vi "HFRR ADV v021 new software.vi"() -> ()   [LabVIEW 2025] (continued)
            n322 = property on="Password 3" class="Clust (strict)"("Visible"=TRUE) -> ()  [unwired: 2 in, 2 out]
            n323 = property on="Service Password Log" class="Str"("Visible"=TRUE) -> ()  [unwired: 2 in, 2 out]
          }
        }
      }
      event "Password 3.Service Password": Value Change {
        n324 = event-data() -> ()  [unwired: 1 in, 6 out]
        n325 = Unbundle By Name("Password 3") -> ("Service Password"=w417:string)
        n326 = call <vilib>:"Trim Whitespace.vi"("string"=w417) -> ("trimmed string"=w415:string)  [unwired: 1 in]
        n327 = Equal?(x=w415, y="Service@123") -> (x = y?=w416:bool)
        n328 = case shown="False" w416 {
          selector: w416 -> [w421 w423]
          frame False {
            n329 = local write "Service Password enable"(w421) -> ()
            n330 = property on="Service Password Log" class="Str"("Visible"=TRUE) -> ()  [unwired: 2 in, 2 out]
            n331 = property on="Tab Control 5" class="TabCtl (strict)"("Tabs Visible?"=TRUE ("Page Labels Display Visible?")) -> ()  [unwired: 2 in, 2 out]
          }
          frame True {
            n332 = property on="Service Password Log" class="Str"("Visible"=FALSE) -> ()  [unwired: 2 in, 2 out]
            "Service Password enable" <- w423
          }
        }
      }
      event "Sign In": Value Change {
        w425 = FALSE ("Visible")
        n333 = event-data() -> ()  [unwired: 1 in, 6 out]
        n334 = property on="About" class="Clust (strict)"("Visible"=w425) -> ()  [unwired: 2 in, 2 out]
        n335 = property on="Password 3" class="Clust (strict)"("Visible"=w425) -> ()  [unwired: 2 in, 2 out]
        n336 = property on="Service Password Log" class="Str"("Visible"=FALSE) -> ()  [unwired: 2 in, 2 out]
      }
      event "Info": Value Change {
        n337 = event-data() -> ()  [unwired: 1 in, 6 out]
        n338 = local read "Info"() -> (w427:bool)
        n339 = case shown="False" w427 {
          frame False {
            n340 = property on="About" class="Clust (strict)"("Visible"=FALSE) -> ()  [unwired: 2 in, 2 out]
          }
          frame True {
            n341 = property on="About" class="Clust (strict)"("Visible"=TRUE) -> ()  [unwired: 2 in, 2 out]
          }
        }
      }
      event "Calibration": Value Change {
        n342 = event-data() -> ()  [unwired: 1 in, 6 out]
        n343 = local read "Calibration"() -> (w431:bool)
        n344 = case shown="False" w431 {
          frame False {
            n345 = property on="Calibration 2" class="TabCtl (strict)"("Visible"=FALSE) -> ()  [unwired: 2 in, 2 out]
            n346 = local write "Cal Password"("" ("Cal Password")) -> ()
          }
          frame True {
            n347 = property on="Calibration 2" class="TabCtl (strict)"("Visible"=TRUE) -> ()  [unwired: 2 in, 2 out]
            n348 = local write "Cal Password"("" ("Cal Password")) -> ()
          }
        }
        n349 = property on="Wrong Password" class="Str"("Visible"=FALSE) -> ()  [unwired: 2 in, 2 out]
      }
      event "Cal Password": Value Change {
        n350 = event-data() -> ()  [unwired: 1 in, 6 out]
        n351 = local read "Cal Password"() -> (w439:string)
        n352 = call <vilib>:"Trim Whitespace.vi"("string"=w439) -> ("trimmed string"=w438:string)  [unwired: 1 in]
        n353 = Equal?(x=w438, y="Cal@321") -> (x = y?=w436:bool)
        n354 = case shown="True" w436 {
          frame False {
            n355 = property on="Wrong Password" class="Str"("Visible"=TRUE) -> ()  [unwired: 2 in, 2 out]
          }
          frame True {
            n356 = property on="Wrong Password" class="Str"("Visible"=FALSE) -> ()  [unwired: 2 in, 2 out]
            n357 = local write "Main Tab"(T2."About" ("Main Tab")) -> ()
            n358 = local write "Cal Password"("" ("Cal Password")) -> ()
            n359 = local write "Main Dashboard Buttons"(T1."About" ("Main Dashboard Buttons")) -> ()
            n360 = local write "Tab Control 5"(T12."Temperature Calibration" ("Tab Control 5")) -> ()
            n361 = property on="Calibration 2" class="TabCtl (strict)"("Visible"=FALSE) -> ()  [unwired: 2 in, 2 out]
            n362 = property on="Tab Control 5" class="TabCtl (strict)"("Tabs Visible?"=FALSE ("Page Labels Display Visible?")) -> ()  [unwired: 2 in, 2 out]
            n363 = local write "Calibration"(FALSE ("Calibration")) -> ()
          }
        }
      }
      event "Calibration Selection": Value Change {
        n364 = event-data() -> ()  [unwired: 1 in, 6 out]
        n365 = local read "Calibration Selection"() -> (w450:T8)
        n366 = case shown="\"Stroke Calibration\"" w450 {
          tunnel: [T7."Stroke" ("Main Calibration Tab") T7."Friction" ("Main Calibration Tab") T7."Main" ("Main Calibration Tab") T7."Temperature" ("Main Calibration Tab")] -> w449
          frame "Stroke Calibration" {
          }
          frame "Friction Force Calibration" {
          }
          frame Default {
          }
          frame "Temperature Calibration" {
          }
        }
        n367 = local write "Main Calibration Tab"(w449) -> ()
      }
      event "Back Stroke": Value Change {
        n368 = event-data() -> ()  [unwired: 1 in, 6 out]
        n369 = local write "Main Stroke Tab"(T9."Step 1" ("Main Stroke Tab")) -> ()
        n370 = local write "Main Calibration Tab"(T7."Main" ("Main Calibration Tab")) -> ()
        n371 = local write "Back Stroke"(FALSE ("Back Stroke")) -> ()
      }
      event "Step 2 Back": Value Change {
        n372 = event-data() -> ()  [unwired: 1 in, 6 out]
        n373 = local write "Main Stroke Tab"(T9."Step 1" ("Main Stroke Tab")) -> ()
        n374 = local write "Step 2 Back"(FALSE ("Back Stroke")) -> ()
      }
      event "Step 3 Back": Value Change {
        n375 = event-data() -> ()  [unwired: 1 in, 6 out]
        n376 = local write "Main Stroke Tab"(T9."Step 2" ("Main Stroke Tab")) -> ()
        n377 = local write "Step 3 Back"(FALSE ("Back Stroke")) -> ()
      }
      event "Step 4 Back": Value Change {
        n378 = event-data() -> ()  [unwired: 1 in, 6 out]
        n379 = local write "Main Stroke Tab"(T9."Step 3" ("Main Stroke Tab")) -> ()
        n380 = local write "Step 4 Back"(FALSE ("Back Stroke")) -> ()
      }
      event "Step 5 Back": Value Change {
        n381 = event-data() -> ()  [unwired: 1 in, 6 out]
        n382 = local write "Main Stroke Tab"(T9."Step 4" ("Main Stroke Tab")) -> ()
        n383 = local write "Step 5 Back"(FALSE ("Back Stroke")) -> ()
      }
      event "Step 6 Back": Value Change {
        n384 = event-data() -> ()  [unwired: 1 in, 6 out]
        n385 = local write "Main Stroke Tab"(T9."Step 5" ("Main Stroke Tab")) -> ()
        n386 = local write "Step 6 Back"(FALSE ("Back Stroke")) -> ()
      }
      event "Back Stroke step 7": Value Change {
        n387 = event-data() -> ()  [unwired: 1 in, 6 out]
        n388 = local write "Main Stroke Tab"(T9."Step 6" ("Main Stroke Tab")) -> ()
        n389 = local write "Back Stroke step 7"(FALSE ("Back Stroke")) -> ()
      }
      event "Back Stroke step 8": Value Change {
        n390 = event-data() -> ()  [unwired: 1 in, 6 out]
        n391 = local write "Main Stroke Tab"(T9."Step 7" ("Main Stroke Tab")) -> ()
        n392 = local write "Back Stroke step 8"(FALSE ("Back Stroke")) -> ()
      }
      event "Back Stroke 8": Value Change {
        n393 = event-data() -> ()  [unwired: 1 in, 6 out]
        n394 = local write "MOVE CARRIAGE TO"(0.2 ("MOVE CARRIAGE TO")) -> ()
        n395 = local write "Main Stroke Tab"(T9."Step 1" ("Main Stroke Tab")) -> ()
        n396 = local write "Back Stroke 8"(FALSE ("Back Stroke 8")) -> ()
      }
      event "Continue Stroke": Value Change {
        n397 = event-data() -> ()  [unwired: 1 in, 6 out]
        n398 = local write "Main Stroke Tab"(T9."Step 2" ("Main Stroke Tab")) -> ()
        n399 = local write "Continue Stroke"(FALSE ("Continue Stroke")) -> ()
      }
      event "Continue Stroke step 2": Value Change {
        n400 = event-data() -> ()  [unwired: 1 in, 6 out]
        n401 = local write "Main Stroke Tab"(T9."Step 3" ("Main Stroke Tab")) -> ()
        n402 = local write "Continue Stroke step 2"(FALSE ("Continue Stroke")) -> ()
      }
      event "Continue Stroke step 3": Value Change {
        n403 = event-data() -> ()  [unwired: 1 in, 6 out]
        n404 = local write "Main Stroke Tab"(T9."Step 4" ("Main Stroke Tab")) -> ()
        n405 = local write "Continue Stroke step 3"(FALSE ("Continue Stroke")) -> ()
      }
      event "Continue Stroke step 4": Value Change {
        n406 = event-data() -> ()  [unwired: 1 in, 6 out]
        n407 = local write "Main Stroke Tab"(T9."Step 5" ("Main Stroke Tab")) -> ()
        n408 = local write "Continue Stroke step 4"(FALSE ("Continue Stroke")) -> ()
      }
      event "Continue Stroke step 5": Value Change {
        n409 = event-data() -> ()  [unwired: 1 in, 6 out]
        n410 = local write "Main Stroke Tab"(T9."Step 6" ("Main Stroke Tab")) -> ()
        n411 = local write "Continue Stroke step 5"(FALSE ("Continue Stroke")) -> ()
      }
      event "Continue Stroke step 6": Value Change {
        n412 = event-data() -> ()  [unwired: 1 in, 6 out]
        n413 = local write "Main Stroke Tab"(T9."Step 7" ("Main Stroke Tab")) -> ()
        n414 = local write "Continue Stroke step 6"(FALSE ("Continue Stroke")) -> ()
      }
      event "Continue Stroke step 7": Value Change {
        w489 = FALSE ("0.2mm")
        n415 = event-data() -> ()  [unwired: 1 in, 6 out]
        n416 = local write "0.4 mm"(w489) -> ()
        n417 = local write "0.6 mm"(w489) -> ()
        n418 = local write "1.0 mm"(w489) -> ()
        n419 = local write "1.2 mm"(w489) -> ()
        n420 = local write "0.2 2"(w489) -> ()
        n421 = local write "0.4 2"(w489) -> ()
        n422 = local write "0.6 2"(w489) -> ()
        n423 = local write "0.8 2"(w489) -> ()
        n424 = local write "1.0 2"(w489) -> ()
        n425 = local write "1.2"(w489) -> ()
        n426 = local write "0.2mm"(w489) -> ()
        n427 = local write "0.8mm"(w489) -> ()
        n428 = local write "Main Stroke Tab"(T9."Step 8" ("Main Stroke Tab")) -> ()
        n429 = local write "Continue Stroke step 7"(FALSE ("Continue Stroke")) -> ()
        n430 = local write "Stroke Test Complete"(T10."Test Progress" ("Stroke Test Complete")) -> ()
        "Position Measurment Temp" <- 0.0 ("Position Measurment Temp")
        "Calibration Tare" <- TRUE ("Calibration Tare")
        "MOVE CARRIAGE TO" <- 0.2 ("MOVE CARRIAGE TO")
      }
      event "Continue Stroke step 8": Value Change {
        n431 = event-data() -> ()  [unwired: 1 in, 6 out]
        n432 = local read "LVDT STROKE  Calibration"() -> (w494:dbl)
        n433 = local read "Position Measurment Temp"() -> (w495:dbl)
        n434 = case shown="4" w495 {
          selector: w495 -> [w500 w505 w510 w515 w520 w524 w527 w528]
          tunnel: w494 -> [w496 w501 w506 w511 w516 w521 _ _]
          frame 0, Default {
            w498 = TRUE ("0.2mm")
            n435 = Increment(x=w500) -> (x+1=w499:i32)
            n436 = local write "Position Measurment Temp"(w499) -> ()
            n437 = local write "0.2mm"(w498) -> ()
            n438 = local write "0.2 2"(w498) -> ()
            n439 = local write "MOVE CARRIAGE TO"(0.4 ("MOVE CARRIAGE TO")) -> ()
            "Calibration 0.2" <- w496
          }
          frame 1 {
            w503 = TRUE ("0.4 mm")
            n440 = Increment(x=w505) -> (x+1=w504:i32)
            n441 = local write "Calibration 0.4"(w501) -> ()
            n442 = local write "Position Measurment Temp"(w504) -> ()
            n443 = local write "0.4 mm"(w503) -> ()
            n444 = local write "MOVE CARRIAGE TO"(0.6 ("MOVE CARRIAGE TO")) -> ()
            n445 = local write "0.4 2"(w503) -> ()
          }
          frame 2 {
            w508 = TRUE ("0.6 mm")
            n446 = Increment(x=w510) -> (x+1=w509:i32)
            n447 = local write "Calibration 0.6"(w506) -> ()
            n448 = local write "Position Measurment Temp"(w509) -> ()
            n449 = local write "0.6 2"(w508) -> ()
            n450 = local write "0.6 mm"(w508) -> ()
            n451 = local write "MOVE CARRIAGE TO"(0.8 ("MOVE CARRIAGE TO")) -> ()
          }
          frame 3 {
            w512 = TRUE ("0.6 mm")
            n452 = Increment(x=w515) -> (x+1=w514:i32)
            n453 = local write "Position Measurment Temp"(w514) -> ()
            n454 = local write "MOVE CARRIAGE TO"(1.0 ("MOVE CARRIAGE TO")) -> ()
            n455 = local write "0.8mm"(w512) -> ()
            n456 = local write "0.8 2"(w512) -> ()
            "Calibration 0.8" <- w511
          }
          frame 4 {
            w517 = TRUE ("0.6 mm")
            n457 = Increment(x=w520) -> (x+1=w519:i32)
            n458 = local write "Position Measurment Temp"(w519) -> ()
            n459 = local write "MOVE CARRIAGE TO"(1.2 ("MOVE CARRIAGE TO")) -> ()
            n460 = local write "1.0 mm"(w517) -> ()
            n461 = local write "1.0 2"(w517) -> ()
            "Calibration 1.0" <- w516
          }
          frame 5 {
            w522 = TRUE ("0.6 mm")
            n462 = Increment(x=w524) -> (x+1=w523:i32)
            n463 = local write "Position Measurment Temp"(w523) -> ()
            n464 = local write "1.2 mm"(w522) -> ()
            n465 = local write "1.2"(w522) -> ()
            "Calibration 1.2" <- w521
          }
          frame 6 {
            n466 = Increment(x=w527) -> (x+1=w526:i32)
            n467 = local write "Position Measurment Temp"(w526) -> ()
            n468 = local write "Stroke Test Complete"(T10."Stroke Points Completed" ("Stroke Test Complete")) -> ()
          }
          frame 7 {
            n469 = stacked-sequence {
              tunnel: w528 -> [w529 _ _]
              frame #0 {
                n470 = Increment(x=w529) -> (x+1=w530:i32)
                n471 = local write "Main Stroke Tab"(T9."Step 9" ("Main Stroke Tab")) -> ()
                n472 = local write "Position Measurment Temp"(w530) -> ()
                n473 = Insert Into Array(array=dbl[] [], new element #1=0.2 ("new element/subarray"), new element #2=0.4 ("new element/subarray"), new element #3=0.6 ("new element/subarray"), new element #4=0.8 ("new element/subarray"), new element #5=1.0 ("new element/subarray"), new element #6=1.2 ("new element/subarray")) -> (→"1D stroke":dbl[])  [unwired: 1 in]
                n474 = local read "Calibration 0.2"() -> (w537:dbl)
                n475 = local read "Calibration 0.4"() -> (w536:dbl)
                n476 = local read "Calibration 0.6"() -> (w535:dbl)
                n477 = local read "Calibration 0.8"() -> (w534:dbl)
                n478 = local read "Calibration 1.0"() -> (w533:dbl)
                n479 = local read "Calibration 1.2"() -> (w532:dbl)
                n480 = Insert Into Array(array=dbl[] [], new element #1=w537, new element #2=w536, new element #3=w535, new element #4=w534, new element #5=w533, new element #6=w532) -> (→"Calibrated Voltage Value":dbl[])  [unwired: 1 in]
              }
              frame #1 {
                n481 = local read "Calibrated Voltage Value"() -> (w549:dbl[])
                n482 = local read "1D stroke"() -> (w550:dbl[])
                n483 = for {
                  tunnel: [w553] -> w548 mode=indexing
                  tunnel: w550 -> [w552] mode=indexing
                  tunnel: w549 -> [w551] mode=indexing
                  n484 = formula code="if (stroke == 0.2) {\n    status = (voltage >= 0.0961 && voltage <= 0.4961) ? 1 : 0;\n} else if (stroke == 0.4) {\n    status = (voltage >= 0.3425 && voltage <= 0.7425) ? 1 : 0;\n} else if (stroke == 0.6) {\n    status = (voltage >= 0.5370 && voltage <= 0.9370) ? 1 : 0;\n} else if (stroke == 0.8) {\n    status = (voltage >= 0.6640 && voltage <= 1.0640) ? 1 : 0;\n} else if (stroke == 1.0) {\n    status = (voltage >= 0.9000 && voltage <= 1.1000) ? 1 : 0;\n} else if (stroke == 1.2) {\n    status = (voltage >= 0.9278 && voltage <= 1.3278) ? 1 : 0;\n} else {\n    status = 0; // Fails if an invalid stroke value is supplied\n}"("stroke"=w552, "voltage"=w551) -> ("status"=w553:dbl)
                }
                "Status" <- w548
              }
              frame #2 {
                w560 = 1.0
                n485 = local read "Status"() -> (w567:dbl[])
                n486 = Index Array(array=w567) -> (element #1=w566:dbl, element #2=w565:dbl, element #3=w564:dbl, element #4=w563:dbl, element #5=w562:dbl, element #6=w561:dbl)  [unwired: 6 in]
                n487 = Equal?(x=w565, y=w560) -> (x = y?=w558:bool)
                n488 = Equal?(x=w564, y=w560) -> (x = y?=w557:bool)
                n489 = Equal?(x=w563, y=w560) -> (x = y?=w556:bool)
                n490 = Equal?(x=w562, y=w560) -> (x = y?=w555:bool)
                n491 = Equal?(x=w561, y=w560) -> (x = y?=w554:bool)
                n492 = Equal?(x=w566, y=w560) -> (x = y?=w559:bool)
                n493 = case shown="True" w559 {
                  selector: w559 -> [w578 w579]
                  frame True {
                    n494 = local write "Point 1 - 0.2 mm"(w578) -> ()
                    n495 = property on="Point 1 - 0.2 mm" class="Bool"("Caption.Visible"=w578) -> ()  [unwired: 2 in, 2 out]
                  }
                  frame False {
                    n496 = local write "Point 1 - 0.2 mm"(w579) -> ()
                    n497 = property on="Point 1 - 0.2 mm" class="Bool"("Caption.Visible"=w579) -> ()  [unwired: 2 in, 2 out]
                  }
                }
                n498 = case shown="True" w558 {
                  selector: w558 -> [w576 w577]
                  frame True {
                    n499 = local write "Point 2 - 0.4 mm"(w576) -> ()
                    n500 = property on="Point 2 - 0.4 mm" class="Bool"("Caption.Visible"=w576) -> ()  [unwired: 2 in, 2 out]
                  }
                  frame False {
                    n501 = local write "Point 2 - 0.4 mm"(w577) -> ()
                    n502 = property on="Point 2 - 0.4 mm" class="Bool"("Caption.Visible"=w577) -> ()  [unwired: 2 in, 2 out]
                  }
                }
                n503 = case shown="True" w555 {
                  selector: w555 -> [w570 w571]
                  frame True {
                    n504 = local write "Point 5 - 1.0 mm"(w570) -> ()
                    n505 = property on="Point 5 - 1.0 mm" class="Bool"("Caption.Visible"=w570) -> ()  [unwired: 2 in, 2 out]
                  }
                  frame False {
                    n506 = local write "Point 5 - 1.0 mm"(w571) -> ()
                    n507 = property on="Point 5 - 1.0 mm" class="Bool"("Caption.Visible"=w571) -> ()  [unwired: 2 in, 2 out]
                  }
                }
                n508 = case shown="True" w557 {
                  selector: w557 -> [w574 w575]
                  frame True {
                    n509 = local write "Point 3 - 0.6 mm"(w574) -> ()
                    n510 = property on="Point 3 - 0.6 mm" class="Bool"("Caption.Visible"=w574) -> ()  [unwired: 2 in, 2 out]
                  }
                  frame False {
                    n511 = local write "Point 3 - 0.6 mm"(w575) -> ()
                    n512 = property on="Point 3 - 0.6 mm" class="Bool"("Caption.Visible"=w575) -> ()  [unwired: 2 in, 2 out]
                  }
                }
                n513 = case shown="True" w556 {
                  selector: w556 -> [w572 w573]
                  frame True {
                    n514 = local write "Point 4 - 0.8 mm"(w572) -> ()
                    n515 = property on="Point 4 - 0.8 mm" class="Bool"("Caption.Visible"=w572) -> ()  [unwired: 2 in, 2 out]
                  }
                  frame False {
                    n516 = local write "Point 4 - 0.8 mm"(w573) -> ()
                    n517 = property on="Point 4 - 0.8 mm" class="Bool"("Caption.Visible"=w573) -> ()  [unwired: 2 in, 2 out]
                  }
                }
                n518 = case shown="True" w554 {
                  selector: w554 -> [w568 w569]
                  frame True {
                    n519 = local write "Point 6 - 1.2 mm"(w568) -> ()
                    n520 = property on="Point 6 - 1.2 mm" class="Bool"("Caption.Visible"=w568) -> ()  [unwired: 2 in, 2 out]
                  }
                  frame False {
                    n521 = local write "Point 6 - 1.2 mm"(w569) -> ()
                    n522 = property on="Point 6 - 1.2 mm" class="Bool"("Caption.Visible"=w569) -> ()  [unwired: 2 in, 2 out]
                  }
                }
              }
            }
          }
        }
      }
      event "TEMPERATURE STEP Back 1", "TEMPERATURE STEP Back air Temp": Value Change {
        n523 = event-data() -> ()  [unwired: 1 in, 6 out]
        n524 = stacked-sequence {
          frame #0 {
            n525 = local write "Main Calibration Tab"(T7."Main" ("Main Calibration Tab")) -> ()
          }
          frame #1 {
            n526 = Wait (ms)(milliseconds to wait=u32 1000) -> ()  [unwired: 1 out]
          }
          frame #2 {
            n527 = local write "Command"("CAL;END" ("Command")) -> ()
          }
          frame #3 {
            n528 = Wait (ms)(milliseconds to wait=u32 2000) -> ()  [unwired: 1 out]
          }
          frame #4 {
            n529 = local write "Command"("CAL;END" ("Command")) -> ()
          }
        }
      }
      event "Temperature Continue Step 1": Value Change {
        n530 = event-data() -> ()  [unwired: 1 in, 6 out]
        n531 = stacked-sequence {
          frame #0 {
            n532 = Wait (ms)(milliseconds to wait=u32 1500) -> ()  [unwired: 1 out]
          }
          frame #1 {
            n533 = local write "Command"("CAL;START" ("Command")) -> ()
          }
          frame #2 {
            n534 = Wait (ms)(milliseconds to wait=u32 1500) -> ()  [unwired: 1 out]
          }
          frame #3 {
            n535 = local write "Command"("CAL;START" ("Command")) -> ()
          }
          frame #4 {
            n536 = Wait (ms)(milliseconds to wait=u32 2000) -> ()  [unwired: 1 out]
          }
          frame #5 {
          }
          frame #6 {
            n537 = Wait (ms)(milliseconds to wait=u32 2000) -> ()  [unwired: 1 out]
          }
          frame #7 {
            # "CAL;A1;<true_T>"
            n538 = local write "Command"("CAL;A1;0" ("Command")) -> ()
          }
          frame #8 {
            n539 = local write "Tab Control 4"(T11."Step 2" ("Tab Control 4")) -> ()
          }
        }
      }
      event "Temperature Continue Step air Step 1": Value Change {
        n540 = event-data() -> ()  [unwired: 1 in, 6 out]
        n541 = stacked-sequence {
          frame #0 {
            n542 = Wait (ms)(milliseconds to wait=u32 1500) -> ()  [unwired: 1 out]
          }
          frame #1 {
            n543 = local write "Command"("CAL;START" ("Command")) -> ()
          }
          frame #2 {
            n544 = local write "Tab Control 4"(T11."Air Step 2" ("Tab Control 4")) -> ()
            n545 = Wait (ms)(milliseconds to wait=u32 1500) -> ()  [unwired: 1 out]
          }
          frame #3 {
            n546 = local write "Command"("CAL;START" ("Command")) -> ()
          }
          frame #4 {
            n547 = Wait (ms)(milliseconds to wait=u32 2000) -> ()  [unwired: 1 out]
          }
          frame #5 {
            # "CAL;A1;<true_T>"
            n548 = local write "Command"("CAL;A2;0" ("Command")) -> ()
          }
          frame #6 {
            n549 = Wait (ms)(milliseconds to wait=u32 2000) -> ()  [unwired: 1 out]
          }
          frame #7 {
            # "CAL;A1;<true_T>"
            n550 = local write "Command"("CAL;A1;0" ("Command")) -> ()
          }
        }
      }
      event "Temperature Selection": Value Change {
        n551 = event-data() -> ()  [unwired: 1 in, 6 out]
        n552 = local read "Temperature Selection"() -> (w602:enum32{"Air Temperature", "Sample Temperature"})
        n553 = case shown="\"Sample Temperature\"" w602 {
          frame "Air Temperature", Default {
            n554 = local write "Tab Control 4"(T11."Air Step 1" ("Tab Control 4")) -> ()
          }
          frame "Sample Temperature" {
            n555 = local write "Tab Control 4"(T11."Step 1" ("Tab Control 4")) -> ()
          }
        }
      }
      event "Temperature Continue Step 2": Value Change {
        n556 = event-data() -> ()  [unwired: 1 in, 6 out]
        n557 = stacked-sequence {
          frame #0 {
            n558 = stacked-sequence {
              frame #0 {
                n559 = Wait (ms)(milliseconds to wait=u32 1500) -> ()  [unwired: 1 out]
              }
              frame #1 {
                # "CAL;A1;<true_T>"
                n560 = local write "Command"("CAL;A1;0" ("Command")) -> ()
              }
              frame #2 {
                n561 = Wait (ms)(milliseconds to wait=u32 1500) -> ()  [unwired: 1 out]
              }
              frame #3 {
                # "CAL;A1;<true_T>"
                n562 = local write "Command"("CAL;A1;0" ("Command")) -> ()
              }
              frame #4 {
              }
            }
          }
          frame #1 {
            n563 = local write "Tab Control 4"(T11."Step 3" ("Tab Control 4")) -> ()
          }
        }
      }
      event "Temperature Continue Step 3": Value Change {
        n564 = event-data() -> ()  [unwired: 1 in, 6 out]
        n565 = stacked-sequence {
          frame #0 {
            n566 = stacked-sequence {
              frame #0 {
                n567 = Wait (ms)(milliseconds to wait=u32 1500) -> ()  [unwired: 1 out]
              }
              frame #1 {
              }
              frame #2 {
              }
              frame #3 {
                # "CAL;A1;<true_T>"
                n568 = local write "Command"("CAL;A1;60" ("Command")) -> ()
              }
              frame #4 {
                n569 = Wait (ms)(milliseconds to wait=u32 2000) -> ()  [unwired: 1 out]
              }
              frame #5 {
                # "CAL;A1;<true_T>"
                n570 = local write "Command"("CAL;A1;60" ("Command")) -> ()
              }
            }
          }
          frame #1 {
            n571 = Wait (ms)(milliseconds to wait=u32 1000) -> ()  [unwired: 1 out]
          }
          frame #2 {
            n572 = local write "Command"("CAL;SAVE" ("Command")) -> ()
          }
          frame #3 {
            n573 = Wait (ms)(milliseconds to wait=u32 1000) -> ()  [unwired: 1 out]
          }
          frame #4 {
            n574 = local write "Command"("CAL;SAVE" ("Command")) -> ()
          }
          frame #5 {
            n575 = Wait (ms)(milliseconds to wait=u32 1000) -> ()  [unwired: 1 out]
          }
          frame #6 {
            # "CAL;END"
            n576 = local write "Command"("CAL;END" ("Command")) -> ()
          }
          frame #7 {
            n577 = Wait (ms)(milliseconds to wait=u32 1000) -> ()  [unwired: 1 out]
          }
          frame #8 {
            # "CAL;END"
            n578 = local write "Command"("CAL;END" ("Command")) -> ()
          }
          frame #9 {
            n579 = local write "Main Calibration Tab"(T7."Temperature" ("Main Calibration Tab")) -> ()
            n580 = local write "Tab Control 4"(T11."Main" ("Tab Control 4")) -> ()
          }
        }
      }
      event "Back Stroke step main temperature": Value Change {
        n581 = event-data() -> ()  [unwired: 1 in, 6 out]
        n582 = stacked-sequence {
          frame #0 {
            n583 = Wait (ms)(milliseconds to wait=u32 1000) -> ()  [unwired: 1 out]
          }
          frame #1 {
            # "CAL;END"
            n584 = local write "Command"("CAL;END" ("Command")) -> ()
          }
          frame #2 {
            n585 = Wait (ms)(milliseconds to wait=u32 1000) -> ()  [unwired: 1 out]
          }
          frame #3 {
            # "CAL;END"
            n586 = local write "Command"("CAL;END" ("Command")) -> ()
          }
          frame #4 {
            n587 = local write "Main Calibration Tab"(T7."Temperature" ("Main Calibration Tab")) -> ()
            n588 = local write "Tab Control 4"(T11."Main" ("Tab Control 4")) -> ()
          }
        }
      }
      event "Quit": Value Change {
        n589 = event-data() -> ()  [unwired: 1 in, 6 out]
      }
    }
    n590 = Wait (ms)(milliseconds to wait=u32 100) -> ()  [unwired: 1 out]
  }
  n591 = while {
    stop <- w634 stop-if-true
    n592 = local read "Ambient Temperature"() -> (w632:dbl)
    n593 = local read "Sample Temperature"() -> (w631:dbl)
    n594 = local write "Temperature — Live (Set A: 60 °C)"(w631) -> ()
    n595 = local write "Temperature — Live (Set A: 60 °C)"(w631) -> ()
    n596 = local write "Temperature — Live (Set A: 0 °C)"(w632) -> ()
    n597 = local write "Sensor value"(w632) -> ()
    n598 = local write "Sensor value"(w631) -> ()
    n599 = local write "Temperature — Live (Set A: 60 °C)"(w632) -> ()
    n600 = local write "Sensor value"(w631) -> ()
    n601 = local write "Sensor value"(w632) -> ()
    n602 = Wait (ms)(milliseconds to wait=u32 200) -> ()  [unwired: 1 out]
    n603 = local read "Quit"() -> (w634:bool)
  }
  n604 = while {
    shift-right: [w636] -> _
    shift-left: "Enum - Selector" -> [w637]
    stop <- w638 stop-if-true
    # "Auto Start Logic Loop"
    n605 = case shown="\"Humidity & Temperature On\"" w637 {
      tunnel: [w641 w647 w674 w706 w736 Auto_Start_enum."Exit" ("Enum - Selector") Auto_Start_enum."Init" ("Enum - Selector")] -> w636
      frame "Init", Default {
        n606 = local read "Auto Start Test"() -> (w640:bool)
        n607 = Select(t=Auto_Start_enum."Humidity & Temperature On" ("Enum - Selector"), s=w640, f=Auto_Start_enum."Init") -> (s? t:f=w641:T15)
      }
      frame "Humidity & Temperature On" {
        n608 = stacked-sequence {
          tunnel: [_ _ _ _ _ _ Auto_Start_enum."Reach point" ("Enum - Selector")] -> w644
          frame #0 {
            w649 = T19."Disabled and Grayed Out" ("Disabled")
            w650 = TRUE ("Heater Button")
            n609 = property on="Humidity" class="Bool (strict)"("DisabledEnum"=w649) -> ()  [unwired: 2 in, 2 out]
            n610 = property on="Heater Button" class="Bool (strict)"("DisabledEnum"=w649) -> ()  [unwired: 2 in, 2 out]
            n611 = local write "Heater Button"(w650) -> ()
            n612 = local write "Humidity"(w650) -> ()
            n613 = property on="Heater Button" class="Bool (strict)"("Val(Sgnl)"=TRUE ("Value (Signaling)")) -> ()  [unwired: 2 in, 2 out]
          }
          frame #1 {
            n614 = Wait (ms)(milliseconds to wait=u32 3000) -> ()  [unwired: 1 out]
          }
          frame #2 {
            n615 = local read "Set Temp"() -> (w656:dbl)
            n616 = Number To Fractional String(number=w656, precision (6)=i16 2) -> (F-format string=w653:string)  [unwired: 2 in]
            n617 = Concatenate Strings("ST;" ("Command"), w653) -> (w654:string)
            n618 = local write "Command"(w654) -> ()
          }
          frame #3 {
            n619 = Wait (ms)(milliseconds to wait=u32 1500) -> ()  [unwired: 1 out]
          }
          frame #4 {
            (unwired) i16 2 ("precision (6)")
            n620 = local read "WriteHumidity 2"() -> (w658:string[])
            n621 = local read "Set Rh"() -> (w661:dbl)
            n622 = Number To Fractional String(number=w661) -> (F-format string=w662:string)  [unwired: 3 in]
            n623 = Concatenate Strings("M;" ("new element/subarray"), w662) -> (w663:string)
            n624 = local write "Command"("HE;1" ("Command")) -> ()
            n625 = Insert Into Array(array=w658, new element=w663) -> (w659:string[])  [unwired: 1 in]
            n626 = local write "WriteHumidity 2"(w659) -> ()
          }
          frame #5 {
            n627 = Wait (ms)(milliseconds to wait=u32 1500) -> ()  [unwired: 1 out]
          }
          frame #6 {
            w666 = TRUE ("Reach point temp")
            n628 = local write "Reach point Humidity"(w666) -> ()
            n629 = local write "Reach point temp"(w666) -> ()
          }
        }
        n630 = local read "Auto Start Test"() -> (w646:bool)
        n631 = Not(x=w646) -> (.not. x?=w645:bool)
        n632 = Select(t=Auto_Start_enum."close", s=w645, f=w644) -> (s? t:f=w647:T15)
      }
      frame "Reach point" {
        w675 = TRUE ("PAUSE")
        w683 = 1.0 ("y")
        w686 = 1.0 ("y")
        n633 = local read "Set Temp"() -> (w668:dbl)
        n634 = local read "Set Humidity:"() -> (w682:dbl)
        n635 = local read "Humidity ( %RH )"() -> (w687:dbl)
        n636 = Add(x=w668, y=w686) -> (x+y=w685:dbl)
        n637 = Subtract(x=w668, y=w686) -> (x-y=w684:dbl)
        n638 = Add(x=w682, y=w683) -> (x+y=w681:dbl)
        n639 = Subtract(x=w682, y=w683) -> (x-y=w680:dbl)
        n640 = local read "TEMP"() -> (w688:dbl)
        n641 = In Range and Coerce(upper limit=w681, x=w687, lower limit=w680) -> (In Range?=w669:bool)  [unwired: 1 out]
        n642 = In Range and Coerce(upper limit=w685, x=w688, lower limit=w684) -> (In Range?=w670:bool)  [unwired: 1 out]
        n643 = case shown="True" w669 {
          frame False {
          }
          frame True {
            n644 = case shown="True" "Reach point Humidity" {
              selector: "Reach point Humidity" -> [_ w694]
              frame False {
              }
              frame True {
                n645 = local read "EVENT LOG"() -> (w691:string)
                n646 = Not(x=w694) -> (.not. x?=w693:bool)
                n647 = local write "Reach point Humidity"(w693) -> ()
                n648 = call "Event Log.vi"("Content"="Target Humidity reached", "EVENT LOG"=w691) -> ("EVENT LOG"=w692:string)  [unwired: 8 in, 1 out]
                n649 = local write "EVENT LOG"(w692) -> ()
              }
            }
          }
        }
        n650 = case shown="True" w670 {
          frame False {
          }
          frame True {
            n651 = case shown="True" "Reach point temp" {
              selector: "Reach point temp" -> [_ w700]
              frame False {
              }
              frame True {
                n652 = local read "EVENT LOG"() -> (w697:string)
                n653 = Not(x=w700) -> (.not. x?=w699:bool)
                n654 = local write "Reach point temp"(w699) -> ()
                n655 = call "Event Log.vi"("Content"="Target Temperature reached", "EVENT LOG"=w697) -> ("EVENT LOG"=w698:string)  [unwired: 8 in, 1 out]
                n656 = local write "EVENT LOG"(w698) -> ()
              }
            }
          }
        }
        n657 = local read "Auto Start Test"() -> (w673:bool)
        n658 = And(x=w670, y=w669) -> (x .and. y?=w679:bool)
        n659 = Select(t=Auto_Start_enum."Maintain Stage" ("Enum - Selector"), s=w679, f=Auto_Start_enum."Reach point" ("Enum - Selector")) -> (s? t:f=w676:T15)
        n660 = Not(x=w673) -> (.not. x?=w672:bool)
        n661 = Select(t=Auto_Start_enum."close", s=w672, f=w676) -> (s? t:f=w674:T15)
        n662 = call "ELAPSED TIMER VI.vi"("RESET"=w675, "PAUSE"=w675) -> ()  [unwired: 7 in, 3 out]
      }
      frame "Maintain Stage" {
        w715 = 2.0 ("y")
        w714 = 1.0 ("y")
        # "Humidity and  temperatures Set Point  have been reached"
        n663 = local read "Set Temp"() -> (w701:dbl)
        n664 = local read "Set Humidity:"() -> (w718:dbl)
        n665 = local read "Humidity ( %RH )"() -> (w721:dbl)
        n666 = Add(x=w701, y=w714) -> (x+y=w720:dbl)
        n667 = Subtract(x=w701, y=w714) -> (x-y=w719:dbl)
        n668 = local read "TEMP"() -> (w722:dbl)
        n669 = Add(x=w718, y=w715) -> (x+y=w717:dbl)
        n670 = Subtract(x=w718, y=w715) -> (x-y=w716:dbl)
        n671 = In Range and Coerce(upper limit=w720, x=w722, lower limit=w719) -> (In Range?=w713:bool)  [unwired: 1 out]
        n672 = In Range and Coerce(upper limit=w717, x=w721, lower limit=w716) -> (In Range?=w712:bool)  [unwired: 1 out]
        n673 = And(x=w713, y=w712) -> (x .and. y?=w711:bool)
        n674 = Not(x=w711) -> (.not. x?=w710:bool)
        n675 = call "ELAPSED TIMER VI.vi"("TARGET"=60.0, "RESET"=w710, "PAUSE"=FALSE) -> ("ELAPSED INDICATION"=w707:bool)  [unwired: 6 in, 2 out]
        n676 = case shown="True" w707 {
          tunnel: w707 -> [_ w725]
          tunnel: [Auto_Start_enum."Maintain Stage" ("Enum - Selector") w724] -> w705
          frame False {
          }
          frame True {
            n677 = stacked-sequence {
              tunnel: w725 -> [_ _ _ _ _]
              tunnel: [_ _ _ _ Auto_Start_enum."Start Stage" ("Enum - Selector")] -> w724
              frame #0 {
                n678 = local read "EVENT LOG"() -> (w727:string)
                n679 = call "Event Log.vi"("Content"="Humidity and temperature set point has stabilized.", "EVENT LOG"=w727) -> ("EVENT LOG"=w728:string)  [unwired: 8 in, 1 out]
                n680 = local write "EVENT LOG"(w728) -> ()
              }
              frame #1 {
                n681 = Wait (ms)(milliseconds to wait=u32 100) -> ()  [unwired: 1 out]
              }
              frame #2 {
                n682 = local read "EVENT LOG"() -> (w731:string)
                n683 = call "Event Log.vi"("Content"="Auto Test Started", "EVENT LOG"=w731) -> ("EVENT LOG"=w732:string)  [unwired: 8 in, 1 out]
                n684 = local write "EVENT LOG"(w732) -> ()
              }
              frame #3 {
                w733 = TRUE ("RUN")
                n685 = local write "RUN"(w733) -> ()
                n686 = property on="Auto Start Temp" class="Bool (strict)"("Val(Sgnl)"=w733) -> ()  [unwired: 2 in, 2 out]
                "Auto Start Temp" <- w733
              }
              frame #4 {
              }
            }
          }
        }
        n687 = local read "Auto Start Test"() -> (w704:bool)
        n688 = Not(x=w704) -> (.not. x?=w703:bool)
        n689 = Select(t=Auto_Start_enum."close", s=w703, f=w705) -> (s? t:f=w706:T15)
      }
      frame "Start Stage" {
        w735 = TRUE ("PAUSE")
        n690 = local read "Auto Start Test"() -> (w740:bool)
        n691 = Not(x=w740) -> (.not. x?=w739:bool)
        n692 = Select(t=Auto_Start_enum."close" ("Enum - Selector"), s=w739, f=Auto_Start_enum."Start Stage" ("Enum - Selector")) -> (s? t:f=w736:T15)
        n693 = call "ELAPSED TIMER VI.vi"("RESET"=w735, "PAUSE"=w735) -> ()  [unwired: 7 in, 3 out]
      }
      frame "close" {
        w742 = FALSE ("Heater Button")
        n694 = local write "RUN"(w742) -> ()
        n695 = local write "Heater Button"(w742) -> ()
        n696 = local write "Humidity"(w742) -> ()
        n697 = local write "Auto Start Test"(w742) -> ()
        n698 = property on="Heater Button" class="Bool (strict)"("Val(Sgnl)"=FALSE ("Value (Signaling)")) -> ()  [unwired: 2 in, 2 out]
      }
      frame "Exit" {
      }
    }
    n699 = Wait (ms)(milliseconds to wait=u32 100) -> ()  [unwired: 1 out]
    n700 = local read "Quit"() -> (w638:bool)
  }
  n701 = property on="Service Password Log" class="Str"("Visible"=w20) -> ()  [unwired: 2 in, 2 out]
  n702 = property on="Password 3" class="Clust (strict)"("Visible"=w20) -> ()  [unwired: 2 in, 2 out]
  n703 = while {
    stop <- w771 stop-if-true
    w754 = errorcluster {"status"=FALSE, "code"=0, "source"=""} ("error in (no error) 3")
    # "this loop is for manual report generation"
    n704 = local read "Confirm Measrurement"() -> (w753:bool)
    n705 = case shown="True" w753 {
      selector: w753 -> [_ w861]
      tunnel: errorcluster {"status"=FALSE, "code"=0, "source"=""} ("error in (no error) 3") -> [_ w862]
      tunnel: [_ w860] -> _
      frame False {
      }
      frame True {
        n706 = stacked-sequence {
          tunnel: w862 -> [_ w895 _]
          tunnel: w861 -> [_ _ w1002]
          tunnel: [_ w883 _] -> w860
          frame #0 {
            n707 = String To Path(string="C:\\LAB-IQ\\Image Calibrate v01.dcf") -> (path=w865:path)
            n708 = Open/Create/Replace File ("Open File")(file path (use dialog)=w865) -> (refnum out=w866:refnum<file>)  [unwired: 5 in, 2 out]
            n709 = for {
              N: 4 -> [_]
              tunnel: w866 -> [w872]
              i -> [w868]
              n710 = Read from Text File ("Read File")(file (use dialog)=w872) -> (text=w873:string)  [unwired: 3 in, 3 out]
              n711 = String Subset(string=w873, offset (0)=6, length (rest)=10 ("length (rest)")) -> (substring=w869:string)
              n712 = Fract/Exp String To Number(string=w869) -> (number=w867:dbl)  [unwired: 3 in, 1 out]
              n713 = case shown="3" w868 {
                tunnel: w867 -> [w874 w875 _ w876 _]
                frame 0 {
                  n714 = local write "5x Gain"(w874) -> ()
                }
                frame 1 {
                  n715 = local write "10x Gain"(w875) -> ()
                }
                frame 2 {
                }
                frame 3 {
                  n716 = local write "100x gain"(w876) -> ()
                }
                frame 4, Default {
                }
              }
            }
          }
          frame #1 {
            n717 = local read "TEST STANDARD"() -> (w878:T3)
            n718 = case shown="\"ISO 12156\"" w878 {
              tunnel: ["ASTM D6079" "ISO 12156"] -> w877
              frame "ASTM D6079", Default {
              }
              frame "ISO 12156" {
              }
            }
            n719 = call "IMAGE ANALYSIS.vi"("Enum"=POST_ANALYSIS_ENUM."GET MEASUREMENTS", "error in"=w895) -> ("error out"=w902:errorcluster)  [unwired: 8 in, 1 out]
            n720 = local read "Magnification :"() -> (w888:string)
            n721 = call "Stall Data Flow.vim"("value in"=w902, "milliseconds to wait"=u32 1000) -> ("value out"=w901:errorcluster)  [unwired: 1 out]
            n722 = local read "Test File List :"() -> (w899:string)
            n723 = case shown="\"10x\"" w888 {
              tunnel: [w938 w939] -> w886
              frame "5x", Default {
                n724 = local read "5x Gain"() -> (w938:dbl)
              }
              frame "10x" {
                # "5x"
                n725 = local read "10x Gain"() -> (w939:dbl)
              }
            }
            n726 = call "IMAGE ANALYSIS.vi"("Enum"=POST_ANALYSIS_ENUM."READ", "error in"=w901) -> ("error out"=w898:errorcluster, "data out"=w889:string)  [unwired: 8 in]
            n727 = Match Pattern(string=w889, regular expression="\"type\": ") -> (after substring=w893:string)  [unwired: 1 in, 3 out]
            n728 = call "IMAGE PATH CREATION PY.vi"("error in (no error)"=w898, "File Name :"=w899) -> ("error out"=w897:errorcluster, "File Path"=w885:path, "File Path String:"=w880:string)  [unwired: 7 in]
            n729 = Match Pattern(string=w893, regular expression=",") -> (before substring=w879:string)  [unwired: 1 in, 3 out]
            n730 = local read "Calibration Tab"() -> (w882:enum32{"Measrument", "Calibrate"})
            n731 = call "Stall Data Flow.vim"("value in"=w897, "milliseconds to wait"=u32 250) -> ("value out"=w881:errorcluster)  [unwired: 1 out]
            n732 = Equal?(x=w879, y="\"rectangle\"") -> (x = y?=w890:bool)
            n733 = case shown="False" w890 {
              tunnel: w889 -> [w944 w999]
              tunnel: w886 -> [_ w990]
              tunnel: cluster{"major":dbl, "minor":dbl, "average":dbl} {"major"=0.0, "minor"=0.0, "average"=0.0} -> [w942 w986]
              tunnel: [w941 w983] -> w884
              tunnel: w879 -> [w943 _]
              tunnel: w886 -> [w940 _]
              frame False {
                n734 = Equal?(x=w943, y="\"line\"") -> (x = y?=w945:bool)
                n735 = case shown="True" w945 {
                  tunnel: w944 -> [_ w960]
                  tunnel: w942 -> [w947 w959]
                  tunnel: [w947 w957] -> w941
                  tunnel: w940 -> [_ w956]
                  frame False {
                  }
                  frame True {
                    w955 = 0.0 ("Major Axis")
                    n736 = Match Pattern(string=w960, regular expression="\"length_px\":") -> (after substring=w958:string)  [unwired: 1 in, 3 out]
                    n737 = property on="Major Axis" class="DigNum (strict)"("Caption.Text"="") -> ()  [unwired: 2 in, 2 out]
                    n738 = property on="Minor Axis" class="DigNum (strict)"("Caption.Text"="") -> ()  [unwired: 2 in, 2 out]
                    n739 = property on="Average" class="DigNum (strict)"("Caption.Text"="Line") -> ()  [unwired: 2 in, 2 out]
                    n740 = Fract/Exp String To Number(string=w958, default (0 dbl)=0.0 ("default (0 DBL)")) -> (number=w954:dbl)  [unwired: 2 in, 1 out]
                    "Pixel Value" <- w954
                    n741 = Multiply(x=w954, y=w956) -> (x*y=w967:dbl)
                    n742 = Multiply(x=w967, y=1000.0) -> (x*y=w950:dbl)
                    n743 = Divide(x=w950, y=1000.0) -> (x/y=w953:dbl)
                    n744 = local write "Measurment (mm)"(w953) -> ()
                    n745 = Bundle By Name(cluster=w959, "average"=w950) -> (w957:cluster{"major":dbl, "minor":dbl, "average":dbl})
                    n746 = Number To Fractional String(number=w950, precision (6)=i16 1) -> (F-format string=w949:string)  [unwired: 2 in]
                    n747 = local write "Minor Axis"(w955) -> ()
                    n748 = local write "Major Axis"(w955) -> ()
                    n749 = Fract/Exp String To Number(string=w949) -> (number=w948:dbl)  [unwired: 3 in, 1 out]
                    n750 = local write "Average"(w948) -> ()
                  }
                }
              }
              frame True {
                w987 = 1000.0 ("y")
                w993 = 0.0 ("default (0 DBL)")
                n751 = Match Pattern(string=w999, regular expression=" \"width_px\":") -> (after substring=w997:string)  [unwired: 1 in, 3 out]
                n752 = Match Pattern(string=w997, regular expression="\"height_px\":") -> (before substring=w995:string, after substring=w994:string)  [unwired: 1 in, 2 out]
                n753 = Fract/Exp String To Number(string=w995, default (0 dbl)=w993) -> (number=w992:dbl)  [unwired: 2 in, 1 out]
                n754 = Fract/Exp String To Number(string=w994, default (0 dbl)=w993) -> (number=w991:dbl)  [unwired: 2 in, 1 out]
                n755 = Multiply(x=w992, y=w990) -> (x*y=w989:dbl)
                n756 = Multiply(x=w991, y=w990) -> (x*y=w988:dbl)
                n757 = Multiply(x=w989, y=w987) -> (x*y=w973:dbl)
                n758 = Multiply(x=w988, y=w987) -> (x*y=w971:dbl)
                n759 = Add(x=w973, y=w971) -> (x+y=w985:dbl)
                n760 = property on="Major Axis" class="DigNum (strict)"("Caption.Text"="Major Axis") -> ()  [unwired: 2 in, 2 out]
                n761 = property on="Minor Axis" class="DigNum (strict)"("Caption.Text"="Minor Axis") -> ()  [unwired: 2 in, 2 out]
                n762 = property on="Average" class="DigNum (strict)"("Caption.Text"="Average") -> ()  [unwired: 2 in, 2 out]
                n763 = Divide(x=w985, y=2.0) -> (x/y=w969:dbl)
                n764 = Bundle By Name(cluster=w986, "major"=w973, "minor"=w971, "average"=w969) -> (w983:cluster{"major":dbl, "minor":dbl, "average":dbl})
                n765 = Number To Fractional String(number=w971, precision (6)=i16 1) -> (F-format string=w978:string)  [unwired: 2 in]
                n766 = Number To Fractional String(number=w969, precision (6)=i16 1) -> (F-format string=w979:string)  [unwired: 2 in]
                n767 = Number To Fractional String(number=w973, precision (6)=i16 1) -> (F-format string=w977:string)  [unwired: 2 in]
                n768 = Fract/Exp String To Number(string=w978) -> (number=w970:dbl)  [unwired: 3 in, 1 out]
                n769 = Fract/Exp String To Number(string=w979) -> (number=w968:dbl)  [unwired: 3 in, 1 out]
                n770 = Fract/Exp String To Number(string=w977) -> (number=w972:dbl)  [unwired: 3 in, 1 out]
                n771 = local write "Major Axis"(w972) -> ()
                n772 = local write "Average"(w968) -> ()
                n773 = local write "Minor Axis"(w970) -> ()
              }
            }
            n774 = case shown="\"Measrument\", Default" w882 {
              tunnel: w885 -> [w912 _]
              tunnel: w884 -> [w911 _]
              tunnel: [w908 w937] -> w883
              tunnel: w881 -> [w910 w937]
              tunnel: w880 -> [w909 _]
              tunnel: w877 -> [w907 _]
              frame "Measrument", Default {
                n775 = stacked-sequence {
                  tunnel: w912 -> [w930 _]
                  tunnel: w911 -> [w928 _]
                  tunnel: w910 -> [w926 _]
                  tunnel: w909 -> [w925 _]
                  tunnel: [w920 _] -> w908
                  tunnel: w907 -> [w913 _]
                  frame #0 {
                    n776 = call "IMAGE ANALYSIS.vi"("Enum"=POST_ANALYSIS_ENUM."SAVE IMAGE", "error in"=w926, "IMAGE FILE PATH"=w925) -> ("error out"=w924:errorcluster)  [unwired: 7 in, 1 out]
                    n777 = call "Stall Data Flow.vim"("value in"=w924, "milliseconds to wait"=u32 1000) -> ("value out"=w915:errorcluster)  [unwired: 1 out]
                    n778 = local read "Test File List :"() -> (w932:string)
                    n779 = call "IMAGE ANALYSIS.vi"("Enum"=POST_ANALYSIS_ENUM."MINIMIZE UI", "error in"=w915) -> ("error out"=w922:errorcluster)  [unwired: 8 in, 1 out]
                    n780 = Bundle By Name(cluster=T25 {"File Name"="", "Test Method"="", "Operator"="", "Fuel Description"="", "Date and time"=""} ("Main Ref"), "Test Method"=w913, "File Name"=w932) -> (w933:T25)
                    n781 = call "Stall Data Flow.vim"("value in"=w922, "milliseconds to wait"=u32 1500) -> ("value out"=w917:errorcluster)  [unwired: 1 out]
                    n782 = call "duf file read.vi"("error in (no error)"=w917, "Main Ref"=w933) -> ("error out"=w931:errorcluster, "Main Ref 2"=w929:T25)  [unwired: 8 in]
                    n783 = call "DETECTION REPORT for manual.vi"("error in (no error)"=w931, "return value 3"=w928, "Image File Path"=w930, "Main Ref"=w929) -> ("error out"=w927:errorcluster)  [unwired: 7 in]
                    n784 = call <vilib>:"Clear Errors.vi"("error in (no error)"=w927) -> ("error out"=w918:errorcluster)  [unwired: 5 in, 1 out]
                    n785 = call "IMAGE ANALYSIS.vi"("Enum"=POST_ANALYSIS_ENUM."MINIMIZE UI", "error in"=w918) -> ("error out"=w920:errorcluster)  [unwired: 8 in, 1 out]
                  }
                  frame #1 {
                    n786 = local write "Main Tab"(T2."HOME" ("Main Tab")) -> ()
                    n787 = local write "Main Dashboard Buttons"(T1."Home" ("Main Dashboard Buttons")) -> ()
                  }
                }
              }
              frame "Calibrate" {
              }
            }
          }
          frame #2 {
            n788 = Not(x=w1002) -> (.not. x?=w1001:bool)
            n789 = local write "Confirm Measrurement"(w1001) -> ()
            n790 = local read "Calibration Tab"() -> (w1000:enum32{"Measrument", "Calibrate"})
            n791 = case shown="\"Measrument\", Default" w1000 {
              frame "Measrument", Default {
                (unwired) T20."HOME" ("Main Tab")
                n792 = local write "Main Tab"(T2."HOME" ("Main Tab")) -> ()
              }
              frame "Calibrate" {
              }
            }
          }
        }
      }
    }
    n793 = local read "Humidity"() -> (w745:bool)
    n794 = local read "Save Change"() -> (w750:bool)
    n795 = local read "Calibrate"() -> (w751:bool)
    n796 = local read "Auto Start Test"() -> (w746:bool)
    n797 = case shown="True" w751 {
      selector: w751 -> [_ w858]
      frame False {
      }
      frame True {
        n798 = Not(x=w858) -> (.not. x?=w857:bool)
        n799 = local write "Calibrate"(w857) -> ()
        n800 = local write "Calibration Tab"(enum32{"Measrument", "Calibrate"}."Calibrate" ("Calibration Tab")) -> ()
      }
    }
    n801 = case shown="True" w750 {
      selector: w750 -> [_ w802]
      frame False {
      }
      frame True {
        n802 = stacked-sequence {
          tunnel: w802 -> [_ _ _ _ w856]
          frame #0 {
            n803 = call "IMAGE ANALYSIS.vi"("Enum"=POST_ANALYSIS_ENUM."HIDE UI") -> ()  [unwired: 9 in, 2 out]
          }
          frame #1 {
            n804 = local read "100x gain"() -> (w804:dbl)
            n805 = local read "10x Gain"() -> (w805:dbl)
            n806 = local read "5x Gain"() -> (w806:dbl)
            n807 = Number To Fractional String(number=w805, width (-)=i16 4, precision (6)=i16 7) -> (F-format string=w827:string)  [unwired: 1 in]
            n808 = Number To Fractional String(number=0.0, width (-)=i16 4, precision (6)=i16 7) -> (F-format string=w822:string)  [unwired: 1 in]
            n809 = Number To Fractional String(number=w804, width (-)=i16 4, precision (6)=i16 7) -> (F-format string=w810:string)  [unwired: 1 in]
            n810 = Number To Fractional String(number=w806, width (-)=i16 10 ("precision (6)"), precision (6)=i16 7) -> (F-format string=w836:string)  [unwired: 1 in]
            n811 = Concatenate Strings("[CH1]" ("string"), w836, " - 5x Gain" ("string"), "\r") -> (w826:string)
            n812 = Concatenate Strings("[CH2]" ("string"), w827, " - 10x Gain" ("string"), "\r") -> (w825:string)
            n813 = Concatenate Strings("[CH3]" ("string"), w822, " - 20x Gain" ("string"), "\r") -> (w816:string)
            n814 = Concatenate Strings("[CH4]" ("string"), w810, " - 100x Gain" ("string"), "\r") -> (w809:string)
            n815 = String To Path(string="C:\\LAB-IQ\\Image Calibrate v01.dcf") -> (path=w839:path)
            n816 = Concatenate Strings(w826, w825, w816, w809) -> (w824:string)
            n817 = call <vilib>:"Write Characters To File.vi"("append to file? (new file:F)"=FALSE, "character string"=w824, "file path (dialog if empty)"=w839) -> ()  [unwired: 2 in, 1 out]
          }
          frame #2 {
            n818 = String To Path(string="C:\\LAB-IQ\\Image Calibrate v01.dcf") -> (path=w842:path)
            n819 = Open/Create/Replace File ("Open File")(file path (use dialog)=w842) -> (refnum out=w843:refnum<file>)  [unwired: 5 in, 2 out]
            n820 = for {
              N: 4 -> [_]
              tunnel: w843 -> [w849]
              i -> [w845]
              n821 = Read from Text File ("Read File")(file (use dialog)=w849) -> (text=w850:string)  [unwired: 3 in, 3 out]
              n822 = String Subset(string=w850, offset (0)=6, length (rest)=10 ("length (rest)")) -> (substring=w846:string)
              n823 = Fract/Exp String To Number(string=w846) -> (number=w844:dbl)  [unwired: 3 in, 1 out]
              n824 = case shown="3" w845 {
                tunnel: w844 -> [w851 w852 _ w853 _]
                frame 0 {
                  n825 = local write "5x Gain"(w851) -> ()
                }
                frame 1 {
                  n826 = local write "10x Gain"(w852) -> ()
                }
                frame 2 {
                }
                frame 3 {
                  n827 = local write "100x gain"(w853) -> ()
                }
                frame 4, Default {
                }
              }
            }
          }
          frame #3 {
            n828 = call "IMAGE ANALYSIS.vi"("Enum"=POST_ANALYSIS_ENUM."SHOW UI") -> ()  [unwired: 9 in, 2 out]
          }
          frame #4 {
            n829 = Not(x=w856) -> (.not. x?=w855:bool)
            n830 = local write "Save Change"(w855) -> ()
          }
        }
      }
    }
    n831 = case shown="False" w746 {
      tunnel: w745 -> [w772 _]
      frame False {
        n832 = case shown="True" w772 {
          frame False {
          }
          frame True {
            n833 = local read "Set Humidity:"() -> (w776:dbl)
            n834 = local read "Set Humidity:"() -> (w779:dbl)
            n835 = local read "Humidity ( %RH )"() -> (w780:dbl)
            n836 = Subtract(x=w776, y=2.0) -> (x-y=w774:dbl)
            n837 = Add(x=w779, y=2.0) -> (x+y=w775:dbl)
            n838 = In Range and Coerce(upper limit=w775, x=w780, lower limit=w774) -> (In Range?=w773:bool)  [unwired: 1 out]
            n839 = case shown="True" w773 {
              frame False {
              }
              frame True {
                n840 = case shown="True" "Manual Humididty Reached" {
                  selector: "Manual Humididty Reached" -> [_ w783]
                  frame False {
                  }
                  frame True {
                    n841 = Not(x=w783) -> (.not. x?=w782:bool)
                    n842 = local write "Manual Humididty Reached"(w782) -> ()
                    n843 = local read "EVENT LOG"() -> (w785:string)
                    n844 = call "Event Log.vi"("Content"="Target Humidity reached", "EVENT LOG"=w785) -> ("EVENT LOG"=w784:string)  [unwired: 8 in, 1 out]
                    n845 = local write "EVENT LOG"(w784) -> ()
                  }
                }
              }
            }
          }
        }
      }
      frame True {
        n846 = local write "Manual Humididty Reached"(TRUE ("Manual Humididty Reached")) -> ()
      }
    }
    n847 = local read "Cap Live Image"() -> (w766:bool)
    n848 = local read "SCAR MEASURMENT"() -> (w769:enum32{"Auto Scar", "Manual Scar"})
    n849 = Wait (ms)(milliseconds to wait=u32 250) -> ()  [unwired: 1 out]
    n850 = Equal?(x=w769, y=enum32{"Auto Scar", "Manual Scar"}."Manual Scar" ("SCAR MEASURMENT")) -> (x = y?=w767:bool)
    n851 = And(x=w767, y=w766) -> (x .and. y?=w765:bool)
    n852 = case shown="True" w765 {
      selector: w765 -> [_ w1081]
      frame False {
      }
      frame True {
        n853 = stacked-sequence {
          tunnel: [_ _ _ w1096 _] -> _
          tunnel: w1081 -> [_ _ _ _ w1103]
          frame #0 {
            w1082 = 0.0
            n854 = local write "Major Axis"(w1082) -> ()
            n855 = local write "Minor Axis"(w1082) -> ()
            n856 = local write "Average"(w1082) -> ()
          }
          frame #1 {
            n857 = call "CAMERA LIVE FEED FGV.vi"("Enum - Menu"=CAMERA_LIVE_FEED_ENUM."CAMERA MINIMIZE") -> ()  [unwired: 9 in, 2 out]
          }
          frame #2 {
            n858 = local read "FILE 3"() -> (w1090:string)
            n859 = call <vilib>:"Trim Whitespace.vi"("string"="C:\\LAB-IQ\\images\\") -> ("trimmed string"=w1092:string)  [unwired: 1 in]
            n860 = String To Path(string=w1092) -> (path=w1091:path)
            n861 = Concatenate Strings(w1090, ".png" ("string")) -> (w1089:string)
            n862 = Build Path(base path=w1091, name or relative path=w1089) -> (appended path=w1087:path)
            n863 = Path To String(path=w1087) -> (string=w1086:string)
            n864 = call "CAMERA LIVE FEED FGV.vi"("Enum - Menu"=CAMERA_LIVE_FEED_ENUM."CAMERA SAVE", "Image Path"=w1086) -> ("error out"=w1084:errorcluster)  [unwired: 8 in, 1 out]
            n865 = case shown="No Error" w1084 {
              frame No Error {
                n866 = One Button Dialog(message="Image saved successfully") -> ()  [unwired: 1 in, 1 out]
              }
              frame Error {
              }
            }
          }
          frame #3 {
            n867 = call "LIST FILE NAMES.vi"() -> ("error out"=w1098:errorcluster, "filenames"=w1095:string[])  [unwired: 10 in]
            n868 = call "IMAGE ANALYSIS.vi"("Enum"=POST_ANALYSIS_ENUM."SHOW UI", "error in"=w1098) -> ("error out"=w1096:errorcluster)  [unwired: 8 in, 1 out]
            n869 = property on="Test File List :" class="CmbBox"("Strings[]"=w1095) -> ()  [unwired: 2 in, 2 out]
          }
          frame #4 {
            (unwired) T24."Report" ("Main Dashboard Buttons")
            (unwired) T26."Report" ("Main Dashboard Buttons")
            n870 = Not(x=w1103) -> (.not. x?=w1102:bool)
            n871 = local write "Zoom Factore"(0.0 ("Zoom Factore")) -> ()
            n872 = local write "Cap Live Image"(w1102) -> ()
            n873 = local write "Main Tab"(T2."Adv Scar Report" ("Main Tab")) -> ()
            n874 = property on="Cap Live Image" class="Bool (strict)"("BoolText.Text"="Capture Image" ("Boolean Text.Text")) -> ()  [unwired: 2 in, 2 out]
            n875 = local write "Main Dashboard Buttons"(T1."Report" ("Main Dashboard Buttons")) -> ()
          }
        }
      }
    }
    n876 = local read "change Gain"() -> (w749:bool)
    n877 = local read "Back Square"() -> (w748:bool)
    n878 = case shown="True" w749 {
      selector: w749 -> [_ w793]
      frame False {
      }
      frame True {
        n879 = stacked-sequence {
          tunnel: w793 -> [_ w801]
          frame #0 {
            n880 = local read "Actual (µm)"() -> (w797:dbl)
            n881 = local read "Pixel Value"() -> (w796:dbl)
            n882 = local read "Magnification :"() -> (w795:string)
            n883 = Divide(x=w797, y=w796) -> (x/y=w794:dbl)
            n884 = case shown="\"10x\"" w795 {
              tunnel: w794 -> [w798 w799]
              frame "10x" {
                n885 = local write "10x Gain"(w798) -> ()
              }
              frame "5x", Default {
                n886 = local write "5x Gain"(w799) -> ()
              }
            }
          }
          frame #1 {
            n887 = Not(x=w801) -> (.not. x?=w800:bool)
            n888 = local write "change Gain"(w800) -> ()
          }
        }
      }
    }
    n889 = case shown="True" w748 {
      selector: w748 -> [_ w791]
      frame False {
      }
      frame True {
        n890 = Not(x=w791) -> (.not. x?=w790:bool)
        n891 = local write "Back Square"(w790) -> ()
        n892 = local write "Calibration Tab"(enum32{"Measrument", "Calibrate"}."Measrument" ("Calibration Tab")) -> ()
      }
    }
    n893 = local read "Rectangle Tool"() -> (w760:bool)
    n894 = local read "Clear ROI Tool"() -> (w759:bool)
    n895 = local read "Open Image"() -> (w764:bool)
    n896 = local read "line tool"() -> (w761:bool)
    n897 = local read "OUT"() -> (w762:bool)
    n898 = local read "In"() -> (w763:bool)
    n899 = case shown="True" w764 {
      selector: w764 -> [_ w1069]
      tunnel: [w1065 w1071] -> _
      tunnel: w754 -> [w1065 w1070]
      frame False {
      }
      frame True {
        n900 = Not(x=w1069) -> (.not. x?=w1068:bool)
        n901 = local write "Open Image"(w1068) -> ()
        n902 = call "IMAGE ANALYSIS.vi"("Enum"=POST_ANALYSIS_ENUM."HIDE UI", "error in"=w1070) -> ("error out"=w1078:errorcluster)  [unwired: 8 in, 1 out]
